vi "proportional temp controller.vi"() -> ()   [LabVIEW 2018]
panel:
  out "Temp Setting\nError":bool
  out "Gauge":dbl(knob) scale=0.0..10.0
  out "Output Voltage":dbl
  in  "Low Temp":dbl
  in  "Indicated Temp":dbl(slide) scale=50.0..250.0
  in  "High Temp":dbl
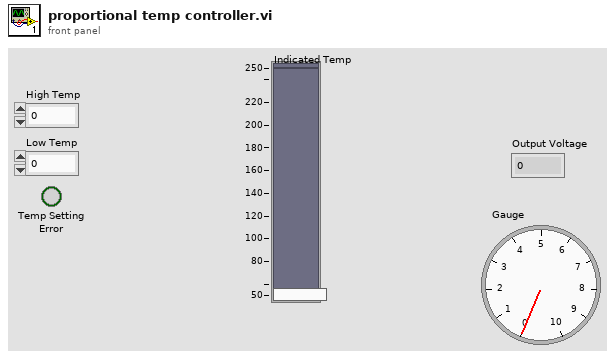
[diagram p1: front panel]
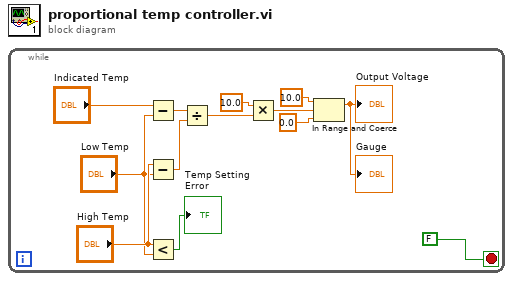
[diagram p0: block diagram]
diagram:
  n1 = while {
    stop <- FALSE stop-if-true
    n2 = Subtract(x="Indicated Temp", y="Low Temp") -> (x-y=w11:dbl)
    n3 = Subtract(x="High Temp", y="Low Temp") -> (x-y=w10:dbl)
    n4 = Less?(x="High Temp", y="Low Temp") -> (x < y?=→"Temp Setting\nError":bool)
    n5 = Divide(x=w11, y=w10) -> (x/y=w9:dbl)
    n6 = Multiply(x=10.0, y=w9) -> (x*y=w4:dbl)
    n7 = In Range and Coerce(upper limit=10.0, x=w4, lower limit=0.0) -> (coerced(x)=→"Output Voltage" →"Gauge":dbl)  [unwired: 1 out]
  }
